vi "Main.vi"(11 "Module Admin":refnum<class "Delacor_lib_QMH_Module Admin.lvclass">) -> ()   [LabVIEW 2020, in "AI DAQ.lvlib"]
doc: "This template is based off of the Queued Message Handler design pattern and the Queued Message Handler project template that ships with LabVIEW.\n\nThe main difference is that the queue is private to this module and communication between modules is performed via Broadcast and Request events.\n\nRequest events are wrapped in public API methods and are handled in the Event Handling Loop (EHL) of this VI. Any module can register for Broadcast events sent by this module. The EHL generates messages based on user interface actions.\n\nThe Message Handling Loop (MHL) processes messages generated by the EHL, or by other messages. The messages are string values, so new messages can be added easily to the Message Cases case structure in the MHL. Each message cluster can also provide an optional value for Message Data, which is a variant that can be converted to whatever message-specific data is required.\n_____\nBased on DQMH Project Template 6.1.0.94."
uses:
  AI DAQ.lvlib
  <vilib>/Delacor/Delacor QMH/Libraries/Module Admin_class/Delacor_lib_QMH_Module Admin.lvclass
  Module Data--cluster.ctl
  <vilib>/Delacor/Delacor QMH/Libraries/Message Queue_class/Delacor_lib_QMH_Message Queue.lvclass/Delacor_lib_QMH_Message Queue.ctl
  Stop Argument--cluster.ctl
  <vilib>/Delacor/Delacor QMH/Libraries/Module Admin_class/Delacor_lib_QMH_Module Admin.lvclass/Delacor_lib_QMH_Module Admin.ctl
  Init AI DAQ Argument--cluster.ctl
  AI DAQ Start Argument--cluster.ctl
  AI DAQ Read Data Argument--cluster.ctl
  AI DAQ Read Data (Reply Payload)--cluster.ctl
  AI DAQ Stop Argument--cluster.ctl
  <vilib>/Utility/miscctls.llb/LVPointTypeDef.ctl
  <vilib>/Delacor/Delacor QMH/Libraries/Message Queue_class/Delacor_lib_QMH_Enqueue Message (Single).vi
  <vilib>/Delacor/Delacor QMH/Libraries/Module Admin_class/Delacor_lib_QMH_Get External Launch.vi
  <vilib>/DAQmx/read.llb/DAQmx Read (Analog 1D Wfm NChan NSamp).vi
  <vilib>/Utility/error.llb/Error Cluster From Error Code.vi
  <vilib>/DAQmx/miscellaneous.llb/DAQmx Fill In Error Info.vi
  <vilib>/ErrorRing/Error Ring.xnode
  <vilib>/Delacor/Delacor QMH/Libraries/Message Queue_class/Delacor_lib_QMH_Message Queue.lvclass
panel:
  out "error out":errorcluster
  out "Status":string
  in  "Simulate MHL Error":bool
  in  "Simulate EHL Error":bool
  # "Other QMH Modules communicate with this Module via its Public API (wrappers for its Request Events).\n\nThis Module communicates with other Modules via its Broadcast Events.\nAny module that wants to get these messages, just registers for this module's Broadcast events."
  # "This template is for the Delacor Modified Queued Message Handler design pattern.\n\nSee the block diagram for more information on how to use this template."
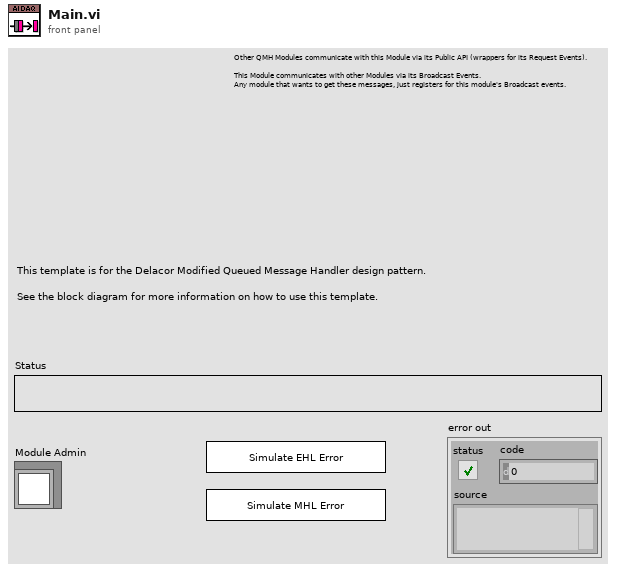
[diagram p1: front panel]
types:
  T1 = typedef "AI DAQ.lvlib/Request Events--cluster.ctl" = cluster{"Stop Module":refnum<user-event>, "Show Panel":refnum<user-event>, "Hide Panel":refnum<user-event>, "Get Module Execution Status":refnum<user-event>, "Show Diagram":refnum<user-event>, "Init AI DAQ":refnum<user-event>, "AI DAQ Start":refnum<user-event>, "AI DAQ Read Data":refnum<user-event>, "AI DAQ Stop":refnum<user-event>}
  T2 = typedef "AI DAQ.lvlib/Module Data--cluster.ctl" = cluster{"Status":string, "AI DAQ Task Name":refnum<k21>}
  T3 = enum32{"invalid lock state", "Not Locked", "Locked (No Password)", "Password-protected"}
  T4 = typedef "AI DAQ.lvlib/Stop Argument--cluster.ctl" = cluster{"Origin":string, "Exit via Stop Module Req?":bool, "Wait for Module to stop?":bool}
  T5 = typedef "AI DAQ.lvlib/Init AI DAQ Argument--cluster.ctl" = cluster{"AI DAQ Task Name":refnum<k21>}
  T6 = typedef "AI DAQ.lvlib/AI DAQ Start Argument--cluster.ctl" = cluster{"Boolean":bool}
  T7 = typedef "AI DAQ.lvlib/AI DAQ Read Data Argument--cluster.ctl" = cluster{"Wait Notifier":refnum<notifier>, "wait for reply":bool}
  T8 = typedef "AI DAQ.lvlib/AI DAQ Stop Argument--cluster.ctl" = cluster{"Boolean":bool}
  T9 = typedef "LVPointTypeDef.ctl" = cluster{"Horizontal":i16, "Vertical":i16}
  T10 = enum32{"Invalid", "Standard", "Closed", "Hidden", "Minimized", "Maximized"}
  T11 = typedef "AI DAQ.lvlib/AI DAQ Read Data (Reply Payload)--cluster.ctl" = cluster{"AI Data Array":waveform(dbl)[], "error":errorcluster}
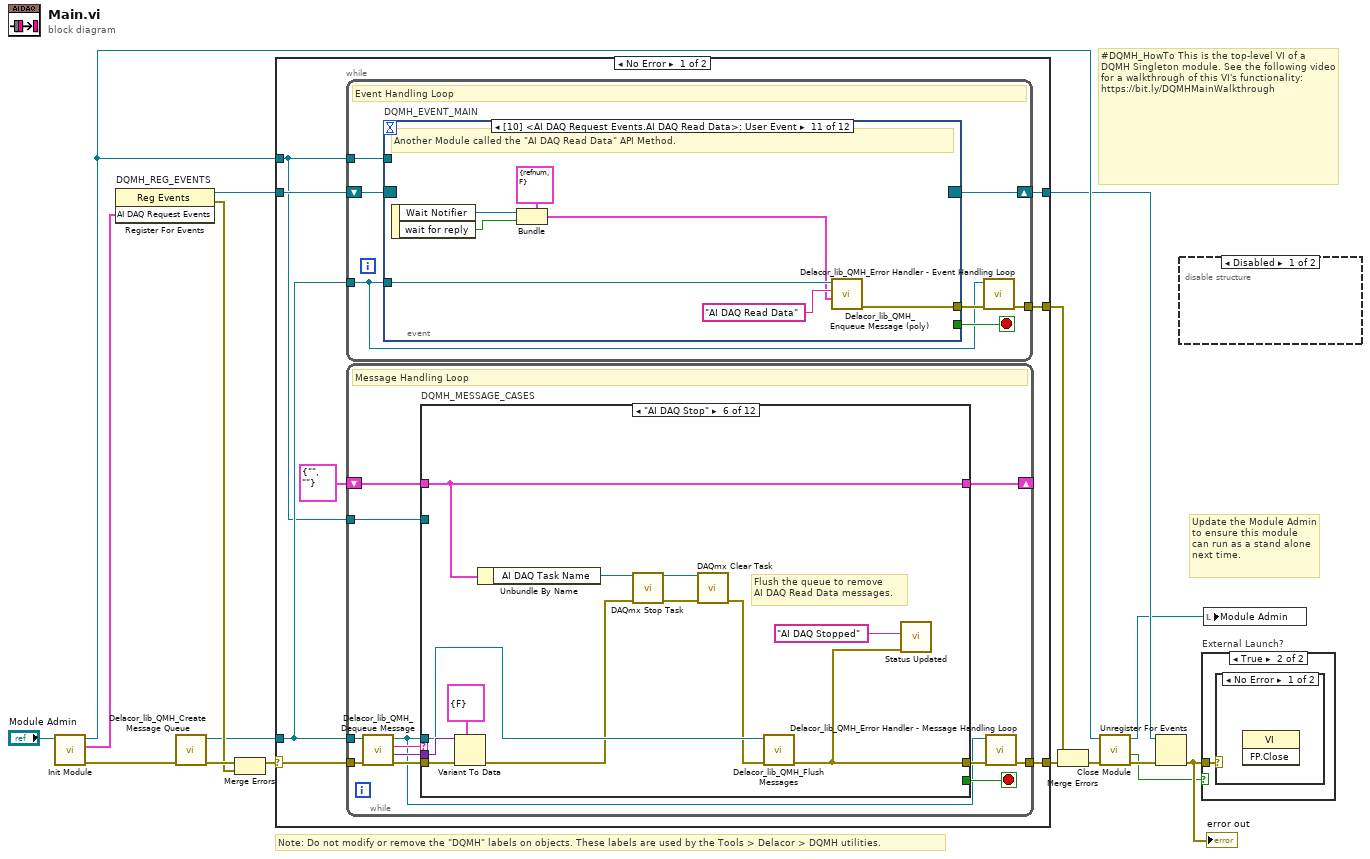
[diagram p0: block diagram]
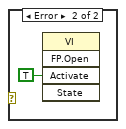
[diagram p4: hidden frame]
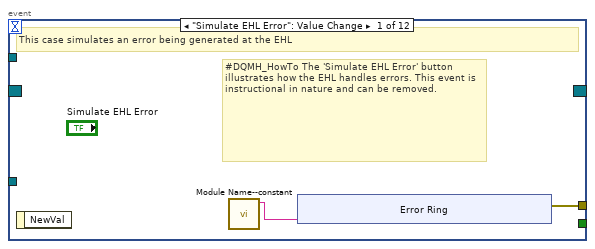
[diagram p5: hidden frame]
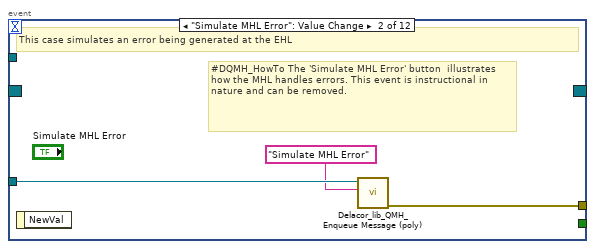
[diagram p6: hidden frame]
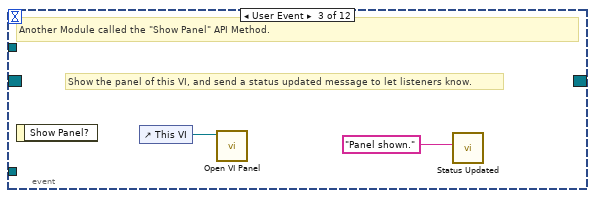
[diagram p7: hidden frame]
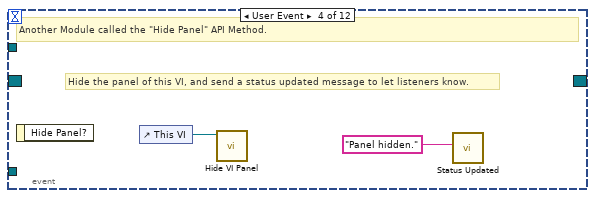
[diagram p8: hidden frame]
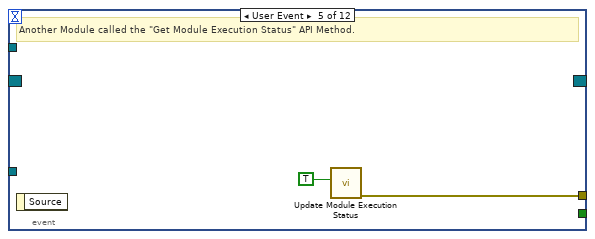
[diagram p9: hidden frame]
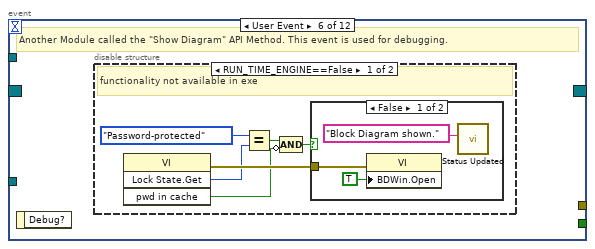
[diagram p10: hidden frame]
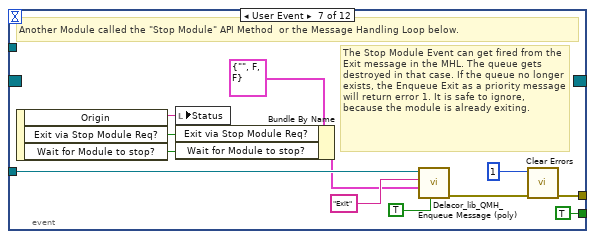
[diagram p13: hidden frame]
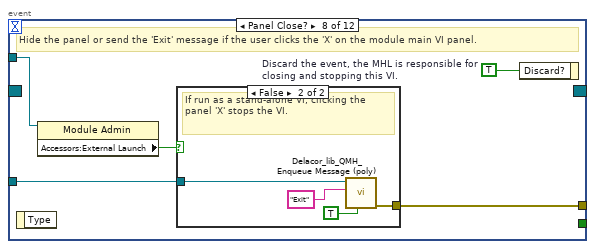
[diagram p14: hidden frame]
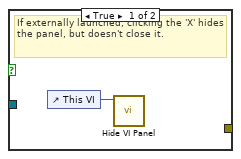
[diagram p15: hidden frame]
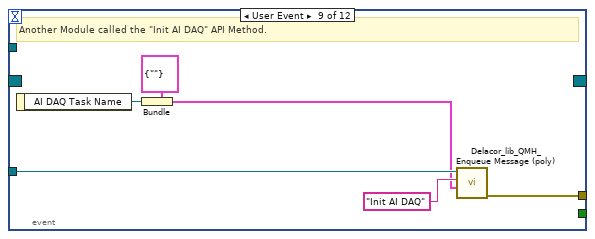
[diagram p16: hidden frame]
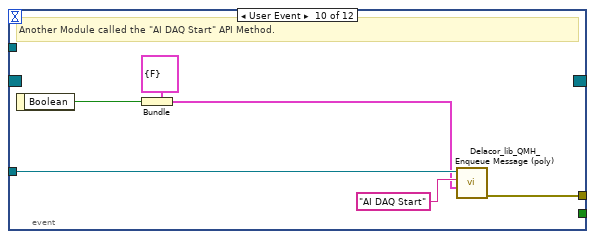
[diagram p17: hidden frame]
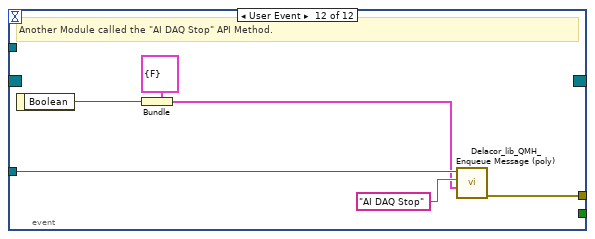
[diagram p18: hidden frame]
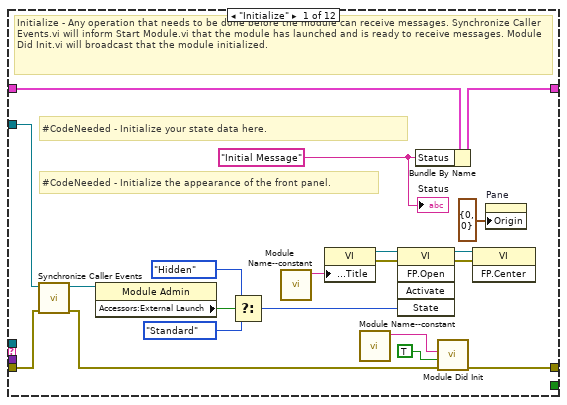
[diagram p19: hidden frame]
diagram:
  # "#DQMH_HowTo This is the top-level VI of a DQMH Singleton module. See the following video for a walkthrough of this VI's functionality: https://bit.ly/DQMHMainWalkthrough"
  # "Note: Do not modify or remove the \"DQMH\" labels on objects. These labels are used by the Tools > Delacor > DQMH utilities."
  # "Update the Module Admin to ensure this module can run as a stand alone next time."
  n1 = call "Init Module.vi"("Singleton Module Admin in"="Module Admin") -> ("error out"=w16:errorcluster, "AI DAQ Request Events"=w5:T1, "Singleton Module Admin out"=w8:refnum<class "Delacor_lib_QMH_Module Admin.lvclass">)  [unwired: 8 in]
  n2 = register-events "DQMH_REG_EVENTS"(w5) -> (reference out=w6:refnum<event-registration>, error out=w9:errorcluster)  [unwired: 2 in]
  n3 = call <vilib>:"Delacor_lib_QMH_Create Message Queue.vi"("error in"=w16) -> ("error out"=w11:errorcluster, "Message Queue"=w4:refnum<class "Delacor_lib_QMH_Message Queue.lvclass">)  [unwired: 9 in]
  n4 = Merge Errors(w11, w9) -> (w10:errorcluster)
  n5 = case shown="No Error" w10 {
    selector: w10 -> [w23 w254]
    tunnel: [w25 w253] -> w17
    tunnel: [w22 w259] -> w7
    tunnel: w6 -> [w20 w259]
    tunnel: w4 -> [w19 w252]
    tunnel: [w24 _] -> w14
    tunnel: w8 -> [w18 w255]
    frame No Error {
      n6 = while {
        tunnel: w19 -> [w26]
        shift-right: [w29] -> w22
        shift-left: w20 -> [w30]
        tunnel: [w31] -> w24
        tunnel: w18 -> [w27]
        stop <- w28 stop-if-true
        # "Event Handling Loop"
        n7 = event "DQMH_EVENT_MAIN" shown="[10] <AI DAQ Request Events.AI DAQ Read Data>: User Event" {
          selector: w30 -> [_ _ _ _ _ _ _ _ _ _ _ _]
          dyn-events: [_ _ _ _ _ _ _ _ _ _ _ _] -> w29
          timeout: _ -> [_ _ _ _ _ _ _ _ _ _ _ _]
          tunnel: [_ _ _ _ _ _ TRUE ("Discard?") _ _ _ _ _] -> w28
          tunnel: w26 -> [_ w43 _ _ _ _ w67 w74 w87 w93 w100 w106]
          tunnel: [w34 w44 _ _ w50 _ w70 w76 w82 w88 w94 w101] -> w32
          tunnel: w27 -> [_ _ _ _ _ _ _ w73 _ _ _ _]
          event "Simulate EHL Error": Value Change {
            # "#DQMH_HowTo The 'Simulate EHL Error' button  illustrates how the EHL handles errors. This event is instructional in nature and can be removed."
            # "This case simulates an error being generated at the EHL"
            n8 = event-data() -> ()  [unwired: 1 in, 1 out]
            n9 = call "Module Name--constant.vi"() -> ("Module Name"=w33:string)  [unwired: 11 in]
            n10 = xnode "Error Ring"("parameter 0"=w33) -> ("error out"=w34:errorcluster)
          }
          event "Simulate MHL Error": Value Change {
            # "#DQMH_HowTo The 'Simulate MHL Error' button  illustrates how the MHL handles errors. This event is instructional in nature and can be removed."
            # "This case simulates an error being generated at the EHL"
            n11 = event-data() -> ()  [unwired: 1 in, 1 out]
            n12 = call-poly <vilib>:"Delacor_lib_QMH_Enqueue Message (poly).vi"("Message"="Simulate MHL Error", "Message Queue in"=w43) -> ("error out"=w44:errorcluster)  [unwired: 8 in, 1 out]
          }
          event User Event {
            # "Show the panel of this VI, and send a status updated message to let listeners know."
            # "Another Module called the \"Show Panel\" API Method."
            n13 = event-data() -> ()  [unwired: 1 in, 1 out]
            n14 = control-ref of="This VI"() -> (w46:refnum<vi>)
            n15 = call "Open VI Panel.vi"("VI"=w46) -> ()  [unwired: 10 in, 1 out]
            n16 = call "Status Updated.vi"("Status"="Panel shown." ("format string")) -> ()  [unwired: 10 in, 1 out]
          }
          event User Event {
            # "Hide the panel of this VI, and send a status updated message to let listeners know."
            # "Another Module called the \"Hide Panel\" API Method."
            n17 = event-data() -> ()  [unwired: 1 in, 1 out]
            n18 = control-ref of="This VI"() -> (w48:refnum<vi>)
            n19 = call "Hide VI Panel.vi"("VI"=w48) -> ()  [unwired: 10 in, 1 out]
            n20 = call "Status Updated.vi"("Status"="Panel hidden." ("format string")) -> ()  [unwired: 10 in, 1 out]
          }
          event User Event {
            # "Another Module called the \"Get Module Execution Status\" API Method."
            n21 = event-data() -> ()  [unwired: 1 in, 1 out]
            n22 = call "Update Module Execution Status.vi"("Running?"=TRUE) -> ("error out"=w50:errorcluster)  [unwired: 10 in]
          }
          event User Event {
            # "Another Module called the \"Show Diagram\" API Method. This event is used for debugging."
            n23 = event-data() -> ()  [unwired: 1 in, 1 out]
            n24 = disable-structure shown="RUN_TIME_ENGINE==False" {
              frame condition #0 (active) {
                # "functionality not available in exe"
                n25 = invoke class="VI" method="Lock State.Get"() -> (error out=w56:errorcluster, "Get Lock State"=w55:T3, "pwd in cache"=w52:bool)  [unwired: 4 in, 1 out]
                n26 = Equal?(x=T3."Password-protected", y=w55) -> (x = y?=w53:bool)
                n27 = Compound Arithmetic op=AND(w53, invert w52) -> (w51:bool)
                n28 = case shown="False" w51 {
                  tunnel: w56 -> [w59 _]
                  frame False {
                    n29 = property class="VI"(error in=w59, "BDWin.Open"=TRUE ("Block Diagram Window:Open")) -> ()  [unwired: 1 in, 2 out]
                    n30 = call "Status Updated.vi"("Status"="Block Diagram shown." ("format string")) -> ()  [unwired: 10 in, 1 out]
                  }
                  frame True {
                    # "Password-protected VI, and the password is not in the cache. Do not show the diagram."
                  }
                }
              }
              frame condition #1 {
              }
            }
          }
          event User Event {
            # "The Stop Module Event can get fired from the Exit message in the MHL. The queue gets destroyed in that case. If the queue no longer exists, the Enqueue Exit as a priority message will return error 1. It is safe to ignore, because the module is already exiting."
            # "Another Module called the \"Stop Module\" API Method  or the Message Handling Loop below."
            n31 = event-data() -> ("Origin"=w66:string, "Exit via Stop Module Req?"=w62:bool, "Wait for Module to stop?"=w61:bool)  [unwired: 1 in]
            n32 = local write "Status"(w66) -> ()
            n33 = Bundle By Name(cluster=T4 {"Origin"="", "Exit via Stop Module Req?"=FALSE, "Wait for Module to stop?"=FALSE} ("Stop Argument"), "Exit via Stop Module Req?"=w62, "Wait for Module to stop?"=w61) -> (w60:T4)
            n34 = call-poly <vilib>:"Delacor_lib_QMH_Enqueue Message (poly).vi"("Priority Message? (F)"=TRUE, "Message Data"=w60, "Message"="Exit", "Message Queue in"=w67) -> ("error out"=w71:errorcluster)  [unwired: 6 in, 1 out]
            n35 = call <vilib>:"Clear Errors.vi"("error in (no error)"=w71, "specific error code to clear (0: all)"=1) -> ("error out"=w70:errorcluster)  [unwired: 4 in, 1 out]
          }
          event Panel Close? {
            w75 = TRUE  # Discard the event, the MHL is responsible for closing and stopping this VI.
            # "Hide the panel or send the 'Exit' message if the user clicks the 'X' on the module main VI panel."
            n36 = event-data() -> ()  [unwired: 1 in, 1 out]
            n37 = property class="Module Admin"(reference=w73) -> ("Accessors:External Launch"=w72:bool)  [unwired: 1 in, 2 out]
            n38 = case shown="False" w72 {
              tunnel: w74 -> [_ w80]
              tunnel: [_ w81] -> w76
              frame True {
                # "If externally launched, clicking the 'X' hides the panel, but doesn't close it."
                n39 = control-ref of="This VI"() -> (w77:refnum<vi>)
                n40 = call "Hide VI Panel.vi"("VI"=w77) -> ()  [unwired: 10 in, 1 out]
              }
              frame False {
                # "If run as a stand-alone VI, clicking the panel 'X' stops the VI."
                n41 = call-poly <vilib>:"Delacor_lib_QMH_Enqueue Message (poly).vi"("Priority Message? (F)"=TRUE, "Message"="Exit", "Message Queue in"=w80) -> ("error out"=w81:errorcluster)  [unwired: 7 in, 1 out]
              }
            }
            n42 = event-data("Discard?"=w75) -> ()  [unwired: 1 in, 1 out]
          }
          event User Event {
            # "Another Module called the \"Init AI DAQ\" API Method."
            n43 = event-data() -> ("AI DAQ Task Name"=w83:refnum<k21>)  [unwired: 1 in]
            n44 = Bundle(cluster=T5 {"AI DAQ Task Name"=""} ("Init AI DAQ Argument"), "AI DAQ Task Name"=w83) -> (w84:T5)
            n45 = call-poly <vilib>:"Delacor_lib_QMH_Enqueue Message (poly).vi"("Message Data"=w84, "Message"="Init AI DAQ", "Message Queue in"=w87) -> ("error out"=w82:errorcluster)  [unwired: 7 in, 1 out]
          }
          event User Event {
            # "Another Module called the \"AI DAQ Start\" API Method."
            n46 = event-data() -> ("Boolean"=w89:bool)  [unwired: 1 in]
            n47 = Bundle(cluster=T6 {"Boolean"=FALSE} ("AI DAQ Start Argument"), "Boolean"=w89) -> (w90:T6)
            n48 = call-poly <vilib>:"Delacor_lib_QMH_Enqueue Message (poly).vi"("Message Data"=w90, "Message"="AI DAQ Start", "Message Queue in"=w93) -> ("error out"=w88:errorcluster)  [unwired: 7 in, 1 out]
          }
          event User Event {
            # "Another Module called the \"AI DAQ Read Data\" API Method."
            n49 = event-data() -> ("Wait Notifier"=w96:refnum<notifier>, "wait for reply"=w95:bool)  [unwired: 1 in]
            n50 = Bundle(cluster=T7 {"Wait Notifier"=refnum, "wait for reply"=FALSE} ("AI DAQ Read Data Argument"), "Wait Notifier"=w96, "wait for reply"=w95) -> (w97:T7)
            n51 = call-poly <vilib>:"Delacor_lib_QMH_Enqueue Message (poly).vi"("Message Data"=w97, "Message"="AI DAQ Read Data", "Message Queue in"=w100) -> ("error out"=w94:errorcluster)  [unwired: 7 in, 1 out]
          }
          event User Event {
            # "Another Module called the \"AI DAQ Stop\" API Method."
            n52 = event-data() -> ("Boolean"=w102:bool)  [unwired: 1 in]
            n53 = Bundle(cluster=T8 {"Boolean"=FALSE} ("AI DAQ Stop Argument"), "Boolean"=w102) -> (w103:T8)
            n54 = call-poly <vilib>:"Delacor_lib_QMH_Enqueue Message (poly).vi"("Message Data"=w103, "Message"="AI DAQ Stop", "Message Queue in"=w106) -> ("error out"=w101:errorcluster)  [unwired: 7 in, 1 out]
          }
        }
        n55 = call-dynamic "Delacor_lib_QMH_Error Handler - Event Handling Loop.vi"("error in"=w32, "Message Queue in"=w26) -> ("dup error in"=w31:errorcluster)  [unwired: 8 in, 1 out]
      }
      n56 = while {
        tunnel: w19 -> [w109]
        shift-right: [w113] -> _
        shift-left: T2 {"Status"="", "AI DAQ Task Name"=""} ("Data Cluster") -> [w114]
        tunnel: w23 -> [w117]
        tunnel: [w115] -> w25
        tunnel: w18 -> [w107]
        stop <- w112 stop-if-true
        # "Message Handling Loop"
        n57 = call-dynamic "Delacor_lib_QMH_Dequeue Message.vi"("error in"=w117, "Message Queue in"=w109) -> ("error out"=w116:errorcluster, "Message Data"=w110:variant, "Message"=w111:string, "Message Queue out"=w108:refnum<class "Delacor_lib_QMH_Message Queue.lvclass">)  [unwired: 6 in]
        n58 = case "DQMH_MESSAGE_CASES" shown="\"AI DAQ Stop\"" w111 {
          selector: w111 -> [_ _ _ _ _ _ _ _ _ _ _ w239]
          tunnel: w108 -> [_ _ _ _ w161 w181 _ _ _ w209 w231 _]
          tunnel: w116 -> [w136 w140 w149 w157 w175 w189 w192 w194 w199 w216 w237 w241]
          tunnel: [w134 w140 w141 w150 w162 w179 w191 w194 w198 w212 w234 w242] -> w118
          tunnel: w114 -> [w125 w139 w145 w154 w168 w186 w190 w193 w196 w211 w230 w240]
          tunnel: [w124 w139 w143 w154 w168 w186 w190 w193 w196 w211 w230 w240] -> w113
          tunnel: [_ _ _ _ _ _ _ _ _ _ w229 _] -> w112
          tunnel: w110 -> [_ _ w148 w156 w159 w188 _ _ _ w210 w228 _]
          tunnel: w107 -> [w126 _ _ _ _ _ _ _ _ w208 w223 _]
          frame "Initialize" {
            w120 = "Initial Message" ("Initial Message")
            # "#CodeNeeded - Initialize the appearance of the front panel."
            # "#CodeNeeded - Initialize your state data here."
            # "Initialize - Any operation that needs to be done before the module can receive messages. Synchronize Caller Events.vi will inform Start Module.vi that the module has launched and is ready to receive messages. Module Did Init.vi will broadcast that the module initialized."
            n59 = call "Synchronize Caller Events.vi"("error in (no error)"=w136, "Singleton Module Admin in"=w126) -> ("error out"=w135:errorcluster, "Singleton Module Admin out"=w121:refnum<class "Delacor_lib_QMH_Module Admin.lvclass">)  [unwired: 8 in]
            n60 = property class="Module Admin"(reference=w121) -> ("Accessors:External Launch"=w130:bool)  [unwired: 1 in, 2 out]
            n61 = Select(t=T10."Hidden" ("State"), s=w130, f=T10."Standard" ("State")) -> (s? t:f=w127:T10)
            n62 = call "Module Name--constant.vi"() -> ("Module Name"=w133:string)  [unwired: 11 in]
            n63 = property class="VI"("Front Panel.Title"=w133) -> (reference out=w132:refnum<vi>, error out=w138:errorcluster)  [unwired: 2 in]
            n64 = call "Module Name--constant.vi"() -> ("Module Name"=w122:string)  [unwired: 11 in]
            n65 = invoke class="VI" method="FP.Open"(reference=w132, error in=w138, "State"=w127) -> (reference out=w131:refnum<vi>, error out=w137:errorcluster)  [unwired: 2 in, 3 out]
            n66 = Bundle By Name(cluster=w125, "Status"=w120) -> (w124:T2)
            n67 = call "Module Did Init.vi"("error in (no error)"=w135, "Initialized?"=TRUE, "Origin"=w122) -> ("error out"=w134:errorcluster)  [unwired: 8 in]
            n68 = invoke class="VI" method="FP.Center"(reference=w131, error in=w137) -> ()  [unwired: 1 in, 3 out]
            n69 = property on="Pane" class="Pane"("Origin"=T9 {"Horizontal"=0, "Vertical"=0}) -> ()  [unwired: 2 in, 2 out]
            "Status" <- w120
          }
          frame "---Module Specific---" {
            # "Separator -- The following cases handle messages specific to this Module."
          }
          frame "Init AI DAQ" {
            # "Initalize the AI DAQ task"
            n70 = Variant To Data(error in=w149, type=T5 {"AI DAQ Task Name"=""} ("Init AI DAQ Argument"), Variant=w148) -> (data=w146:T5, error out=w141:errorcluster)
            n71 = Unbundle By Name(w146) -> ("AI DAQ Task Name"=w144:refnum<k21>)
            n72 = Bundle By Name(cluster=w145, "AI DAQ Task Name"=w144) -> (w143:T2)
            n73 = call "Status Updated.vi"("error in (no error)"=w141, "Status"="Init AI DAQ" ("format string")) -> ()  [unwired: 9 in, 1 out]
          }
          frame "AI DAQ Start" {
            # "Start the AI DAQ task"
            n74 = Unbundle By Name(w154) -> ("AI DAQ Task Name"=w152:refnum<k21>)
            n75 = Variant To Data(error in=w157, type=T6 {"Boolean"=FALSE} ("AI DAQ Start Argument"), Variant=w156) -> (error out=w153:errorcluster)  [unwired: 1 out]
            n76 = call <vilib>:"DAQmx Start Task.vi"("task/channels in"=w152, "error in"=w153) -> ("error out"=w150:errorcluster)  [unwired: 12 in, 1 out]
            n77 = call "Status Updated.vi"("error in (no error)"=w150, "Status"="AI DAQ Start" ("format string")) -> ()  [unwired: 9 in, 1 out]
          }
          frame "AI DAQ Read Data" {
            n78 = Unbundle By Name(w168) -> ("AI DAQ Task Name"=w167:refnum<k21>)
            n79 = Variant To Data(error in=w175, type=T7 {"Wait Notifier"=refnum, "wait for reply"=FALSE} ("AI DAQ Read Data Argument"), Variant=w159) -> (data=w173:T7, error out=w166:errorcluster)
            n80 = Unbundle By Name(w173) -> ("Wait Notifier"=w172:refnum<notifier>, "wait for reply"=w171:bool)
            n81 = call-poly <vilib>:"DAQmx Read.vi"("task/channels in"=w167, "number of samples per channel"=100, "error in"=w166) -> ("data"=w165:waveform(dbl)[], "error out"=w164:errorcluster)  [unwired: 10 in, 1 out]
            n82 = Merge Errors(w166, w164) -> (w163:errorcluster)
            n83 = Bundle By Name(cluster=T11 {"AI Data Array"=[], "error"={"status"=FALSE, "code"=0, "source"=""}} ("AI DAQ Read Data (Reply Payload)"), "AI Data Array"=w165, "error"=w164) -> (w170:T11)
            n84 = case shown="True" w171 {
              tunnel: w172 -> [_ w177]
              tunnel: w170 -> [_ w176]
              frame False {
              }
              frame True {
                n85 = Send Notification(notification=w176, notifier=w177) -> ()  [unwired: 1 in, 2 out]
              }
            }
            n86 = call-poly <vilib>:"Delacor_lib_QMH_Enqueue Message (poly).vi"("error in"=w163, "Message Data"=w159, "Message"="AI DAQ Read Data", "Message Queue in"=w161) -> ("error out"=w162:errorcluster)  [unwired: 6 in, 1 out]
            n87 = call "AI DAQ WF Data.vi"("Reply Payload"=w170) -> ()  [unwired: 10 in, 1 out]
          }
          frame "AI DAQ Stop" {
            # "Flush the queue to remove\nAI DAQ Read Data messages."
            n88 = Variant To Data(error in=w189, type=T8 {"Boolean"=FALSE} ("AI DAQ Stop Argument"), Variant=w188) -> (error out=w180:errorcluster)  [unwired: 1 out]
            n89 = Unbundle By Name(w186) -> ("AI DAQ Task Name"=w184:refnum<k21>)
            n90 = call <vilib>:"DAQmx Stop Task.vi"("task/channels in"=w184, "error in"=w180) -> ("task out"=w183:refnum<k21>, "error out"=w182:errorcluster)  [unwired: 12 in]
            n91 = call <vilib>:"DAQmx Clear Task.vi"("task in"=w183, "error in"=w182) -> ("error out"=w178:errorcluster)  [unwired: 13 in]
            n92 = call-dynamic "Delacor_lib_QMH_Flush Messages.vi"("error in"=w178, "Message Queue in"=w181) -> ("error out"=w179:errorcluster)  [unwired: 6 in, 3 out]
            n93 = call "Status Updated.vi"("error in (no error)"=w179, "Status"="AI DAQ Stopped" ("format string")) -> ()  [unwired: 9 in, 1 out]
          }
          frame "---Copy This Frame---" {
            # "Duplicate this frame when creating new messages.  Change this comment in the duplicated frame to describe this message."
            n94 = Merge Errors(w192) -> (w191:errorcluster)
          }
          frame "---Exit and Error Handling---" {
            # "Separator - The following cases handle errors and exit messages."
          }
          frame "Simulate MHL Error" {
            # "#DQMH_HowTo The 'Simulate MHL Error' button  illustrates how the MHL handles errors. This event is instructional in nature and can be removed."
            # "Simulate an error occurring at the MHL"
            n95 = call "Module Name--constant.vi"() -> ("Module Name"=w195:string)  [unwired: 11 in]
            n96 = xnode "Error Ring"("parameter 0"=w195) -> ("error out"=w197:errorcluster)
            n97 = Merge Errors(w199, w197) -> (w198:errorcluster)
          }
          frame "Error" {
            # "#CodeRecommended - If you ever change the name of this \"Error\" message, you'll need to update the name in the Check Loop Error.vi as well."
            # "#CodeRecommended - If the module is running in standalone mode (External Launch = FALSE), this code will pop up an error dialog and call the 'Exit' message if an error occurs. Add more fine-grained error handling here."
            # "Error - Check the error message data and respond accordingly. This message is sent by the \"Error Handler\" VIs at the end of each loop in this application."
            n98 = property class="Module Admin"(reference=w208) -> ("Accessors:External Launch"=w207:bool)  [unwired: 1 in, 2 out]
            n99 = Variant To Data(error in=w216, type=errorcluster {"status"=FALSE, "code"=0, "source"=""} ("error constant"), Variant=w210) -> (data=w217:errorcluster, error out=w214:errorcluster)
            n100 = call "Error Reported.vi"("Error"=w217) -> ()  [unwired: 10 in, 1 out]
            n101 = case shown="False" w207 {
              tunnel: [w222 _] -> w213
              tunnel: w209 -> [w220 _]
              tunnel: w217 -> [w221 _]
              frame False {
                # "If the module is running standalone, then pop up an error dialog and call the \"Exit\" message."
                n102 = call <vilib>:"Simple Error Handler.vi"("error in (no error)"=w221) -> ()  [unwired: 4 in, 5 out]
                n103 = call-poly <vilib>:"Delacor_lib_QMH_Enqueue Message (poly).vi"("Priority Message? (F)"=TRUE, "Message"="Exit", "Message Queue in"=w220) -> ("error out"=w222:errorcluster)  [unwired: 7 in, 1 out]
              }
              frame True {
                # "If the module was launched externally, calling the Error Reported broadcast VI is the only action performed by the \"Error\" message. The module's caller can then process the error appropriately."
              }
            }
            n104 = Merge Errors(w214, w213) -> (w212:errorcluster)
            n105 = local write "error out"(w212) -> ()
          }
          frame "Exit" {
            w227 = 91  # 91: not all Exit messages will have an argument
            w229 = TRUE  # Stop the VI
            # "Release the message queue reference"
            # "#CodeNeeded - Add any required cleanup code here"
            # "Exit - Exit the application."
            n106 = Variant To Data(error in=w237, type=T4 {"Origin"="", "Exit via Stop Module Req?"=FALSE, "Wait for Module to stop?"=FALSE} ("Stop Argument"), Variant=w228) -> (data=w225:T4, error out=w233:errorcluster)
            n107 = call <vilib>:"Clear Errors.vi"("error in (no error)"=w233, "specific error code to clear (0: all)"=w227) -> ("error out"=w236:errorcluster)  [unwired: 4 in, 1 out]
            n108 = control-ref of="This VI"() -> (w224:refnum<vi>)
            n109 = call-dynamic "Delacor_lib_QMH_Release Message Queue.vi"("error in"=w236, "Message Queue"=w231) -> ("error out"=w235:errorcluster)  [unwired: 9 in]
            n110 = call "Handle Exit.vi"("Stop Argument"=w225, "Admin in"=w223, "VI reference"=w224) -> ("error out"=w232:errorcluster)  [unwired: 7 in, 1 out]
            n111 = Merge Errors(w235, w232) -> (w234:errorcluster)
          }
          frame Default {
            # "'Default' case only runs if there is a message that isn't defined in any of the other cases.  Output a programming error."
            n112 = call "Module Name--constant.vi"() -> ("Module Name"=w238:string)  [unwired: 11 in]
            n113 = xnode "Error Ring"("parameter 0"=w239, "parameter 1"=w238) -> ("error out"=w243:errorcluster)
            n114 = Merge Errors(w241, w243) -> (w242:errorcluster)
          }
        }
        n115 = call-dynamic "Delacor_lib_QMH_Error Handler - Message Handling Loop.vi"("error in"=w118, "Message Queue in"=w108) -> ("dup error in"=w115:errorcluster)  [unwired: 8 in, 1 out]
      }
    }
    frame Error {
      # "Synchronize Caller Events.vi will inform Start Module.vi that the module has launched and will let the code calling Start Module.vi register for broadcasts and would permit the caller receive the broadcast that an error occurred at launch time."
      n116 = call-dynamic "Delacor_lib_QMH_Release Message Queue.vi"("error in"=w254, "Message Queue"=w252) -> ("error out"=w253:errorcluster)  [unwired: 9 in]
      n117 = call "Synchronize Caller Events.vi"("Singleton Module Admin in"=w255) -> ("error out"=w260:errorcluster)  [unwired: 9 in, 1 out]
      n118 = call "Module Name--constant.vi"() -> ("Module Name"=w258:string)  [unwired: 11 in]
      n119 = Format Into String(format string="An error occurred during initialization. %s is no longer running.", w258) -> (resulting string=w256:string)  [unwired: 2 in, 1 out]
      n120 = Merge Errors(w253, w260) -> (w261:errorcluster)
      n121 = call "Error Reported.vi"("Additional Information"=w256, "Error"=w261) -> ()  [unwired: 9 in, 1 out]
    }
  }
  n122 = Merge Errors(w14, w17) -> (w13:errorcluster)
  n123 = call "Close Module.vi"("error in (no error)"=w13, "Module Admin in"=w8) -> ("error out"=w15:errorcluster, "External Launch"=w1:bool, "Module Admin out"=w2:refnum<class "Delacor_lib_QMH_Module Admin.lvclass">)  [unwired: 7 in]
  n124 = Unregister For Events(event registration refnum=w7, error in=w15) -> (error out=w12:errorcluster)
  "error out" <- w12
  n125 = disable-structure shown="Disabled" {
    frame Disabled {
    }
    frame Enabled {
    }
  }
  n126 = case "External Launch?" shown="True" w1 {
    tunnel: w12 -> [_ w262]
    frame False {
    }
    frame True {
      n127 = case shown="No Error" w262 {
        frame No Error {
          n128 = invoke class="VI" method="FP.Close"() -> ()  [unwired: 3 in, 3 out]
        }
        frame Error {
          n129 = invoke class="VI" method="FP.Open"("Activate"=TRUE ("Activate?")) -> ()  [unwired: 4 in, 5 out]
        }
      }
    }
  }
  n130 = local write "Module Admin"(w2) -> ()
